vi "Laser-Commander.vi"(1 "Laser Command":string, 2 "VISA resource name":refnum<visa-resource-name>="Laser") -> (0 "Laser Response":string)   [LabVIEW 2018]
uses:
  <vilib>/Instr/_visa.llb/VISA Configure Serial Port (Instr).vi
panel:
  out "return count":u32
  in  "flow control (0:none)":u16(ring) items=["None", "XON/XOFF", "RTS/CTS", "XON/XOFF & RTS/CTS", "DTR/DSR", "XON/XOFF & DTR/DSR"]
  in  "stop bits (10: 1 bit)":u16(ring)=10 items=["1.0"=10, "1.5"=15, "2.0"=20]
  in  "parity (0:none)":enum16{"None", "Odd", "Even", "Mark", "Space"}(ring)
  in  "data bits (8)":u16=8 min=5 max=8 step=1
  in  "baud rate (9600)":u32=9600
  in  "termination char\n(0xA = '\\n' = LF)":u8=10 format="%.0x"
  in  "Enable Termination\nChar (T)":bool=TRUE
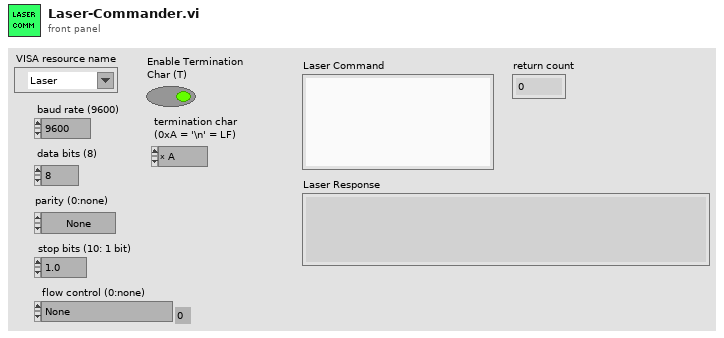
[diagram p1: front panel]
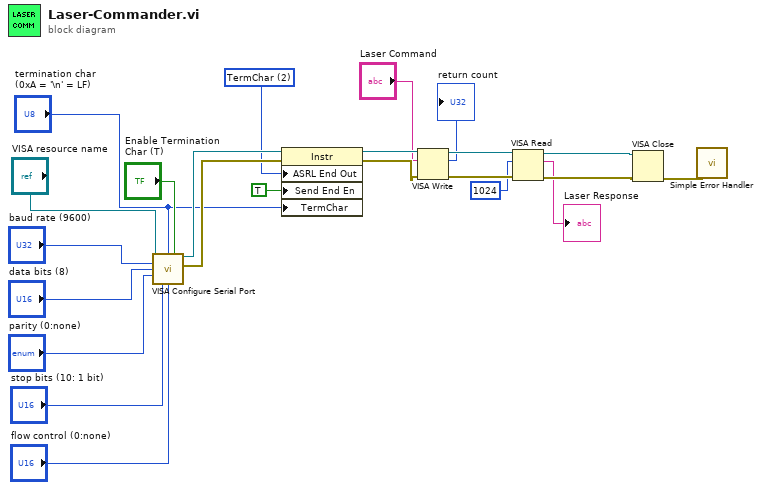
[diagram p0: block diagram]
diagram:
  w14 = u16 2 items=["None", "Last Bit", "TermChar", "Break"] ("Serial Settings:End Mode for Writes")
  n1 = call-poly "VISA Configure Serial Port"("VISA resource name"="VISA resource name", "termination char\n(0xA = '\\n' = LF)"="termination char\n(0xA = '\\n' = LF)", "Enable Termination\nChar (T)"="Enable Termination\nChar (T)", "baud rate (9600)"="baud rate (9600)", "data bits (8)"="data bits (8)", "parity (0:none)"="parity (0:none)", "stop bits (10: 1 bit)"="stop bits (10: 1 bit)", "flow control (0:none)"="flow control (0:none)") -> ("VISA resource name out"=w23:refnum<visa-resource-name>, "error out"=w22:errorcluster)  [unwired: 6 in]
  n2 = property class="Instr"(reference=w23, error in=w22, "ASRL End Out"=w14, "Send End En"=TRUE, "TermChar"="termination char\n(0xA = '\\n' = LF)") -> (reference out=w21:refnum<visa-resource-name>, error out=w20:errorcluster)
  n3 = VISA Write(VISA resource name=w21, write buffer="Laser Command", error in (no error)=w20) -> (VISA resource name out=w19:refnum<visa-resource-name>, return count=→"return count":u32, error out=w17:errorcluster)
  n4 = VISA Read(VISA resource name=w19, byte count=u32 1024, error in (no error)=w17) -> (VISA resource name out=w18:refnum<visa-resource-name>, read buffer=→"Laser Response":string, error out=w16:errorcluster)  [unwired: 1 out]
  n5 = VISA Close(VISA resource name=w18, error in (no error)=w16) -> (error out=w15:errorcluster)
  n6 = call <vilib>:"Simple Error Handler.vi"("error in (no error)"=w15) -> ()  [unwired: 4 in, 5 out]
